vi "Creators Is Created Event.vi"(10 "Created Event Alias":string, 11 "Event in":refnum<class "Event.lvclass">) -> (2 "Is Created Event?":bool, 3 "Event out":refnum<class "Event.lvclass">)   [LabVIEW 2021, in "jettl.lvlib" / "Event.lvclass"]
uses:
  Event.lvclass
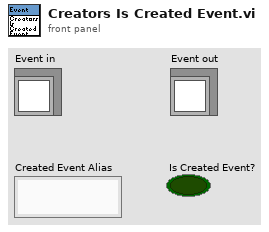
[diagram p1: front panel]
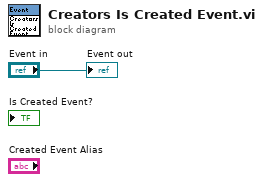
[diagram p0: block diagram]
diagram:
  "Event out" <- "Event in"
